vi "write_params.vi"(8 "error in (no error)":errorcluster, 10 "params":T1={"radius"=1.0, "weights"="uniform", "algorithm"="auto", "leaf_size"=30.0, "p"=2.0, "metric"="minkowski", "outlier_label"={"outlier_label_type"="None", "outlier_label_str"="outlier", "outlier_label_int"=-1.0, "outlier_label_list"=[]}, "n_jobs"=1.0}, 11 "RadiusNeighborsClassifier in":refnum<class "RadiusNeighborsClassifier.lvclass">) -> (0 "error out":errorcluster, 3 "RadiusNeighborsClassifier out":refnum<class "RadiusNeighborsClassifier.lvclass">)   [LabVIEW 2020, in "RadiusNeighborsClassifier.lvclass"]
uses:
  RadiusNeighborsClassifier.lvclass
  Controls/radius_neighbors_classifier_params.ctl
  RadiusNeighborsClassifier.lvclass/RadiusNeighborsClassifier.ctl
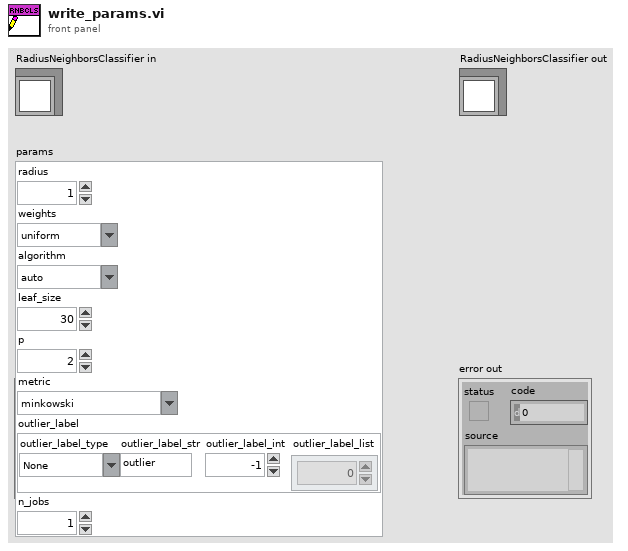
[diagram p1: front panel]
types:
  T1 = typedef "radius_neighbors_classifier_params.ctl" = cluster{"radius":dbl, "weights":string, "algorithm":string, "leaf_size":dbl, "p":dbl, "metric":string, "outlier_label":cluster{"outlier_label_type":string, "outlier_label_str":string, "outlier_label_int":dbl, "outlier_label_list":dbl[]}, "n_jobs":dbl}
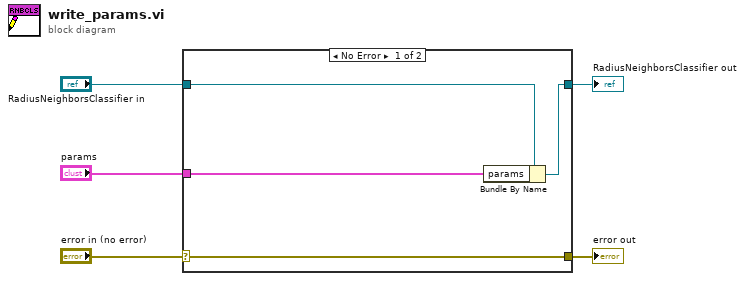
[diagram p0: block diagram]
diagram:
  n1 = case shown="No Error" "error in (no error)" {
    selector: "error in (no error)" -> [w9 w10]
    tunnel: [w9 w10] -> w4
    tunnel: [w7 w11] -> w2
    tunnel: "RadiusNeighborsClassifier in" -> [w8 w11]
    tunnel: "params" -> [w6 _]
    frame No Error {
      n2 = Bundle By Name(cluster=w8, "params"=w6) -> (w7:refnum<class "RadiusNeighborsClassifier.lvclass">)
    }
    frame Error {
    }
  }
  "error out" <- w4
  "RadiusNeighborsClassifier out" <- w2
